vi "Speed.vi"(10 "Speed":i32=20) -> (2 "速度":string)   [LabVIEW 2017]
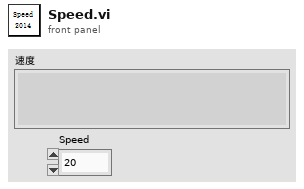
[diagram p1: front panel]
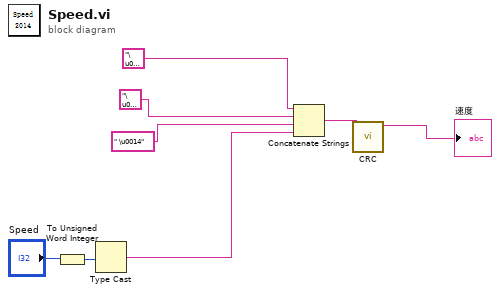
[diagram p0: block diagram]
diagram:
  n1 = To Unsigned Word Integer(number="Speed") -> (unsigned 16bit integer=w1:u16)
  n2 = Type Cast(x=w1) -> (*(type *) &x=w8:string)  [unwired: 1 in]
  n3 = Concatenate Strings("\u0001", "\u0006", " \u0014", w8) -> (w6:string)
  n4 = call "CRC.vi"("字符串"=w6) -> ("连接的字符串"=→"速度":string)  [unwired: 9 in, 1 out]
